vi "Select File Subset.vi"(8 "error in":errorcluster, 11 "Directory":path=path "C:/Users/Christian/Documents") -> (0 "error out":errorcluster, 2 "File List":string[](array[string]))   [LabVIEW 2019]
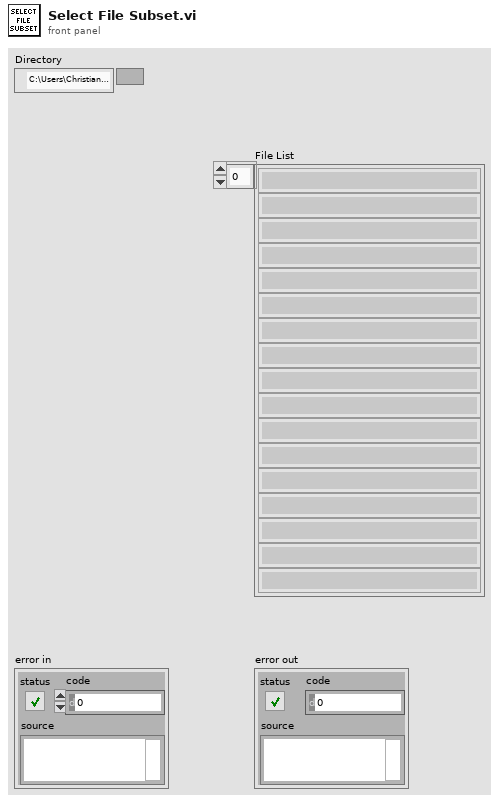
[diagram p1: front panel]
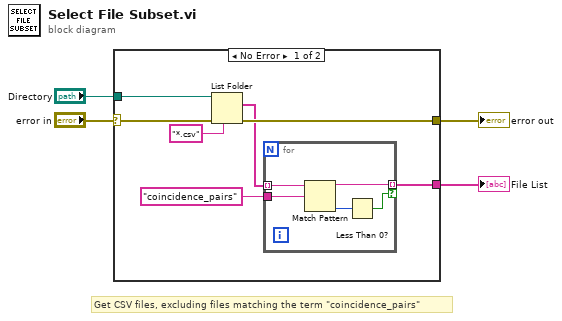
[diagram p0: block diagram]
diagram:
  # "Get CSV files, excluding files matching the term \"coincidence_pairs\""
  n1 = case shown="No Error" "error in" {
    selector: "error in" -> [w5 w17]
    tunnel: "Directory" -> [w10 _]
    tunnel: [w9 w17] -> w3
    tunnel: [w6 _] -> w2
    frame No Error {
      n2 = List Folder(path=w10, pattern="*.csv", error in=w5) -> (filenames=w8:string[], error out=w9:errorcluster)  [unwired: 1 in, 2 out]
      n3 = for {
        tunnel: w8 -> [w16] mode=indexing
        tunnel: "coincidence_pairs" ("regular expression") -> [w15]
        tunnel: [w14] -> w6 mode=indexing if=w13
        n4 = Match Pattern(string=w16, regular expression=w15) -> (before substring=w14:string, offset past match=w12:i32)  [unwired: 1 in, 2 out]
        n5 = Less Than 0?(x=w12) -> (x < 0?=w13:bool)
      }
    }
    frame Error {
    }
  }
  "error out" <- w3
  "File List" <- w2
